vi "Initialize_Control.vi"(0 "GEA2":refnum<queue>, 1 "ERD Loop":refnum<queue>, 5 "Receive Loop Error":refnum<user-event>, 9 "DAQ":refnum<queue>, 11 "Error In":errorcluster, 12 "Cont Send":refnum<queue>) -> (15 "Error Out":errorcluster)   [LabVIEW 2016]
uses:
  type defs/DAQ_States.ctl
  type defs/ERD_Data_Loop_Control.ctl
  type defs/ERD_Data_Loop_States.ctl
  Common/GExplorer Support/typedefs/GExplorer_Data_Cluster.ctl
  type defs/Cont_Send_States.ctl
  type defs/Error_Command.ctl
  type defs/ERD_Loop_Control_Command.ctl
  type defs/GEA2_Control_Command.ctl
  type defs/DAQ_Control_Command.ctl
  type defs/Cont_Send_Loop_Control_Command.ctl
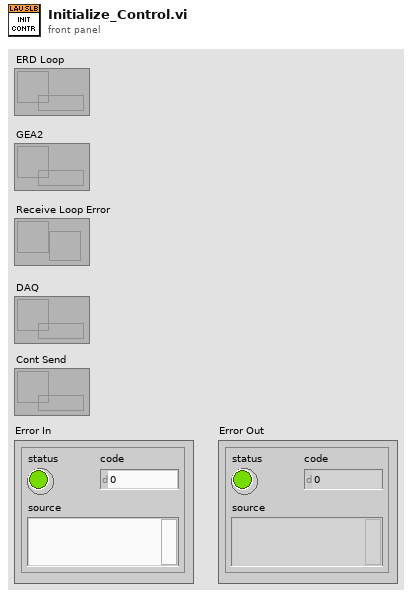
[diagram p1: front panel]
types:
  T1 = typedef "Cont_Send_Loop_Control_Command.ctl" = enum16{"Initialize", "Shutdown"}
  T2 = typedef "DAQ_Control_Command.ctl" = enum16{"Initialize", "Shutdown"}
  T3 = typedef "GEA2_Control_Command.ctl" = enum16{"Initialize", "Shutdown"}
  T4 = typedef "ERD_Loop_Control_Command.ctl" = enum16{"Initialize", "Shutdown"}
  T5 = typedef "Error_Command.ctl" = enum16{"Initialize", "Handle Errors", "Report Errors"}
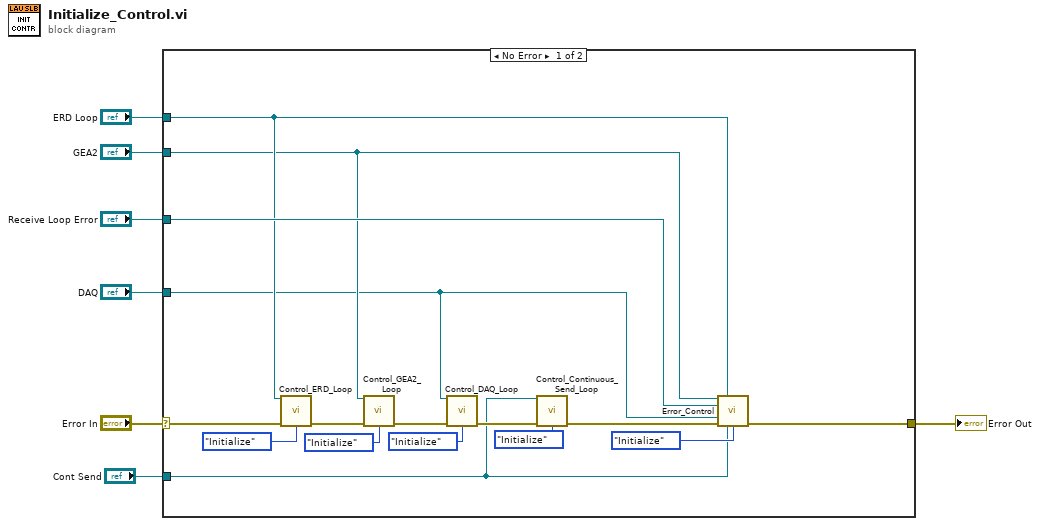
[diagram p0: block diagram]
diagram:
  n1 = case shown="No Error" "Error In" {
    selector: "Error In" -> [w20 w24]
    tunnel: [w23 w24] -> w6
    tunnel: "Receive Loop Error" -> [w22 _]
    tunnel: "ERD Loop" -> [w19 _]
    tunnel: "GEA2" -> [w16 _]
    tunnel: "DAQ" -> [w13 _]
    tunnel: "Cont Send" -> [w8 _]
    frame No Error {
      n2 = call "Control_ERD_Loop.vi"("ERD Loop"=w19, "Command (ERD Loop Control)"=ERD_Loop_Control_Command."Initialize", "Error In"=w20) -> ("Error Out"=w17:errorcluster)  [unwired: 12 in]
      n3 = call "Control_GEA2_Loop.vi"("GEA2"=w16, "Command (ERD Loop Control)"=GEA2_Control_Command."Initialize", "Error In"=w17) -> ("Error Out"=w14:errorcluster)  [unwired: 12 in]
      n4 = call "Control_DAQ_Loop.vi"("DAQ"=w13, "Command (DAQ Control)"=DAQ_Control_Command."Initialize" ("Command (DAQ)"), "Error In"=w14) -> ("Error Out"=w11:errorcluster)  [unwired: 12 in]
      n5 = call "Control_Continuous_Send_Loop.vi"("Cont Send"=w8, "Cont Send Loop Control Command"=Cont_Send_Loop_Control_Command."Initialize", "Error In"=w11) -> ("Error Out"=w10:errorcluster)  [unwired: 12 in]
      n6 = call "Error_Control.vi"("GEA2"=w16, "ERD Loop"=w19, "Command (Handle Errors)"=Error_Command."Initialize", "Loop Error"=w22, "DAQ"=w13, "Error In"=w10, "Cont Send"=w8) -> ("Error Out"=w23:errorcluster)  [unwired: 8 in]
    }
    frame Error {
    }
  }
  "Error Out" <- w6
